vi "NI6071E_HostMain.vi"() -> ()   [LabVIEW 2014, in "NI6071E.lvlib"]
doc: "This VI was developed to test the PH_PPMA_DAQ RT Server Application.\n\nPlease use the PH_PPMA_DAQClient Class within the CS framework."
uses:
  NI6071E.lvlib
  NI6071ECommand.ctl
  NI6071ECommandCluster.ctl
  NI6071EStart.ctl
  NI6071ERead.ctl
  NI6071EConfig.ctl
panel:
  in  "NI6071E DAQ Config RT Client 1":T1={"device (1)"=1, "channels (0)"=["1", "2", "3", "4", "5", "6", "7", "16", "17", "18", "19", "20", "21", "22", "23", "32", "33", "34", "35", "36", "37", "38", "39", "48", "49", "50", "51", "52", "53", "54"], "buffer size (1000 scans)"=1000, "[number of buffers] (1)"=1, "measurement mode structure"={"measurement mode"=0, "reserved"=0}, "input limits (no change)"=[], "coupling & input config (no change:0)"=[{"coupling (no change:0)"=enum."no change", "input config (no change:0)"=1}]} {"measurement mode structure"."measurement mode" items=["no change", "Volts", "Volts RMS", "Ohms", "Diode", "4-wire ohms", "Current", "Current RMS"]; "coupling & input config (no change:0)"."input config (no change:0)" items=["no change", "differential", "ref. single-ended", "non-ref. single-ended", "4-wire"]; "input limits (no change)"."low limit (0.0)" format="%0.2f"; "input limits (no change)"."high limit (0.0)" format="%0.2f"}
  in  "NI6071E DAQ Read":T2={"time limit in sec (-1:auto calculate)"=-1.0, "number of scans to read (-1:all)"=-1} {"time limit in sec (-1:auto calculate)" format="%0.2f"}
  in  "NI6071E DAQ Start":T3={"scan rate (40000 scans/sec)"=1000.0, "trigger type (analog)"=enum."no trigger", "edge or slope \n(rising)"=enum."no change", "number of buffers to acquire (1)"=1, "analog chan (PFI0) & level (2.00)"={"trigger channel (empty)"="", "level (0.0)"=0.0}, "[additional trig params]"={"hysteresis (0.0)"=-1.0, "coupling (no change:0)"=enum."no change", "delay (0 sec)"=0.0, "skip count (0)"=0, "time limit (0 sec)"=0.0}} {"[additional trig params]"."time limit (0 sec)" format="%0.2f"; "[additional trig params]"."delay (0 sec)" format="%0.2f"; "[additional trig params]"."hysteresis (0.0)" format="%0.2f"; "analog chan (PFI0) & level (2.00)"."level (0.0)" format="%0.2f"; "scan rate (40000 scans/sec)" format="%0.2f"}
  out "Measurement":waveform(dbl)[](graph) caption="Measurement data"
  out "RT Error":errorcluster
  in  "NI6071E Command Cluster":T4
  in  "Reset Error":bool
  out "error out":errorcluster
  in  "stop":bool
  out "Response":string
  in  "Connect":bool
  in  "NI6071E DAQ Server":string="apepc01.gsi.de"
  in  "NI6071E Command":T5=enum."CloseConnection"
  in  "Port":u16=6341
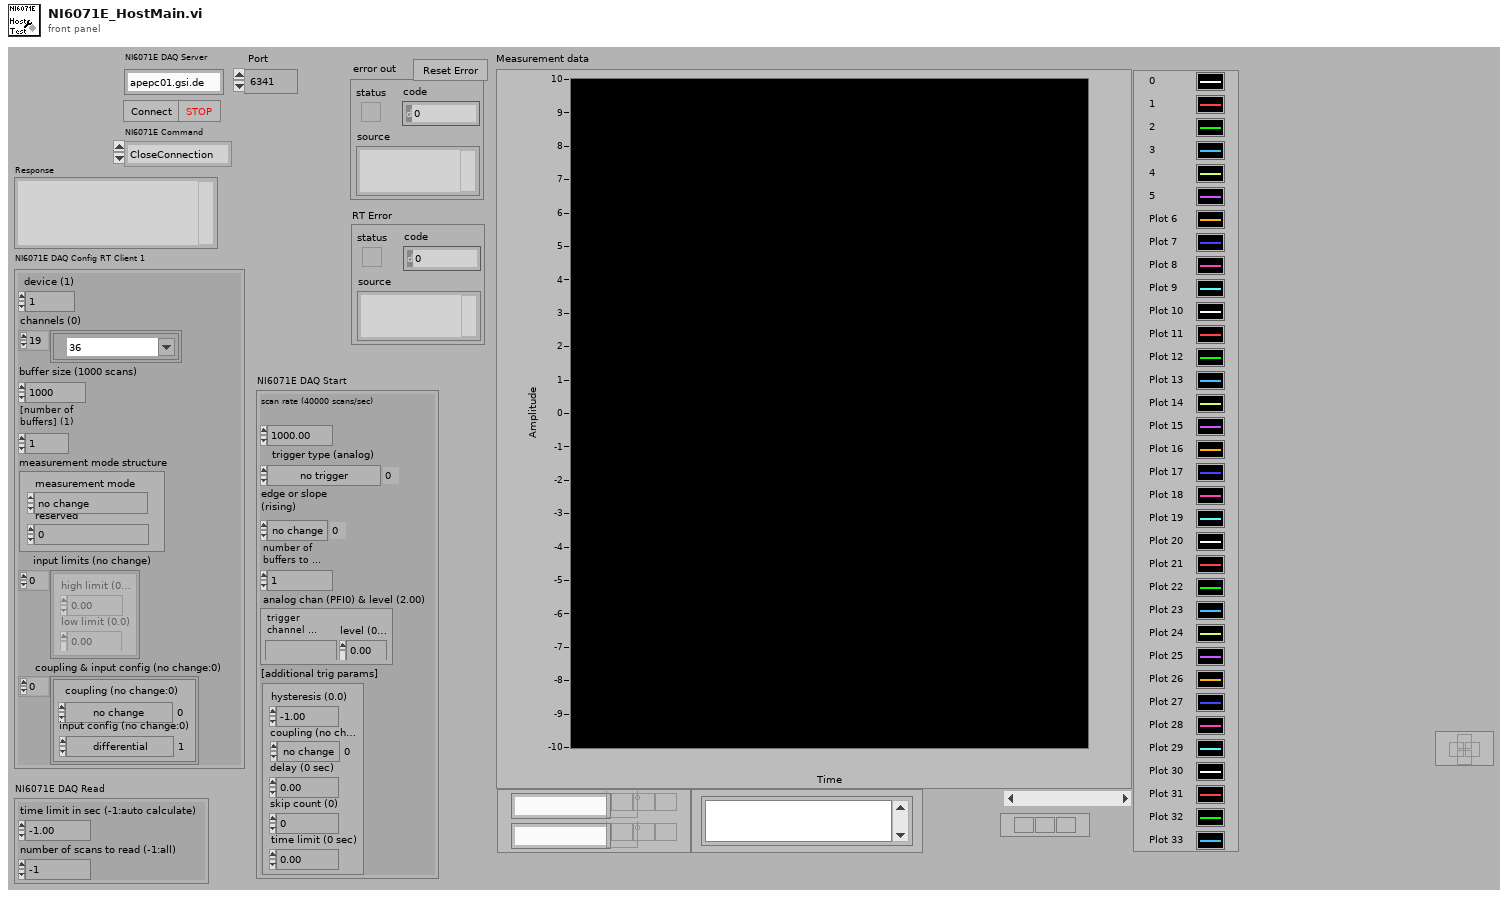
[diagram p1: front panel]
types:
  T1 = typedef "NI6071E.lvlib/NI6071EConfig.ctl" = cluster{"device (1)":i16, "channels (0)":tag[], "buffer size (1000 scans)":i32, "[number of buffers] (1)":i32, "measurement mode structure":cluster{"measurement mode":u16, "reserved":u32}, "input limits (no change)":cluster{"high limit (0.0)":sgl, "low limit (0.0)":sgl}[], "coupling & input config (no change:0)":cluster{"coupling (no change:0)":enum16{"no change", "DC", "AC", "GND", "internal ref."}, "input config (no change:0)":u16}[]}
  T2 = typedef "NI6071E.lvlib/NI6071ERead.ctl" = cluster{"time limit in sec (-1:auto calculate)":sgl, "number of scans to read (-1:all)":i32}
  T3 = typedef "NI6071E.lvlib/NI6071EStart.ctl" = cluster{"scan rate (40000 scans/sec)":sgl, "trigger type (analog)":enum16{"no trigger", "analog", "digital A", "digital A & B", "scan clock gate"}, "edge or slope \n(rising)":enum16{"no change", "rising", "falling"}, "number of buffers to acquire (1)":i32, "analog chan (PFI0) & level (2.00)":cluster{"trigger channel (empty)":string, "level (0.0)":sgl}, "[additional trig params]":cluster{"hysteresis (0.0)":sgl, "coupling (no change:0)":enum16{"no change", "DC", "AC"}, "delay (0 sec)":sgl, "skip count (0)":i32, "time limit (0 sec)":sgl}}
  T4 = typedef "NI6071E.lvlib/NI6071ECommandCluster.ctl" = cluster{"Command":string, "Data":string, "error out":errorcluster}
  T5 = typedef "NI6071E.lvlib/NI6071ECommand.ctl" = enum16{"Ping", "Reset", "ConfigureDAQ", "StartDAQ", "StopDAQ", "GetDAQStatus", "ReadData", "SaveData", "CloseConnection"}
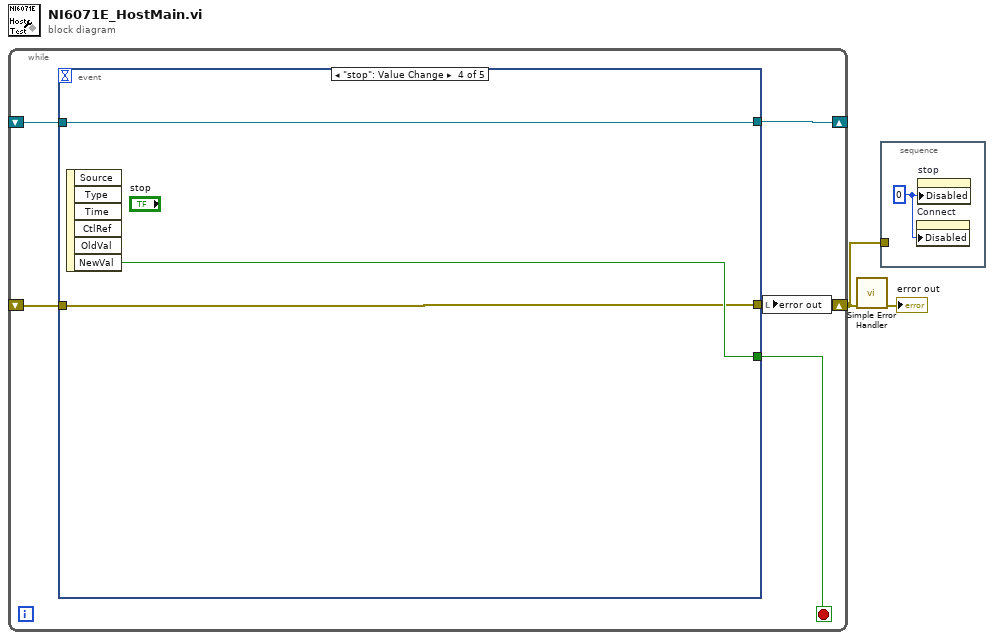
[diagram p0: block diagram]
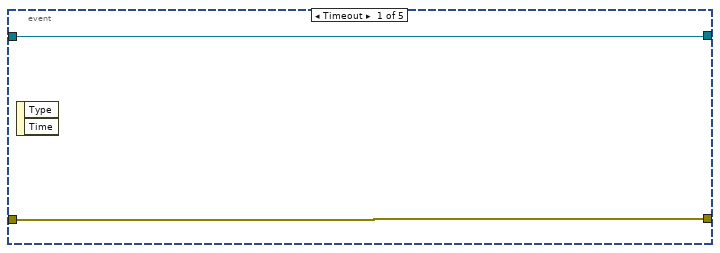
[diagram p2: hidden frame]
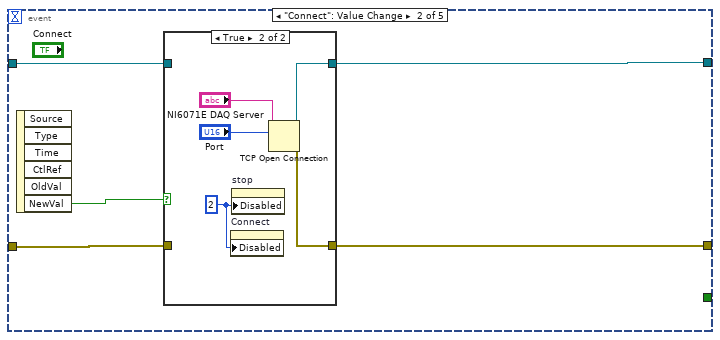
[diagram p3: hidden frame]
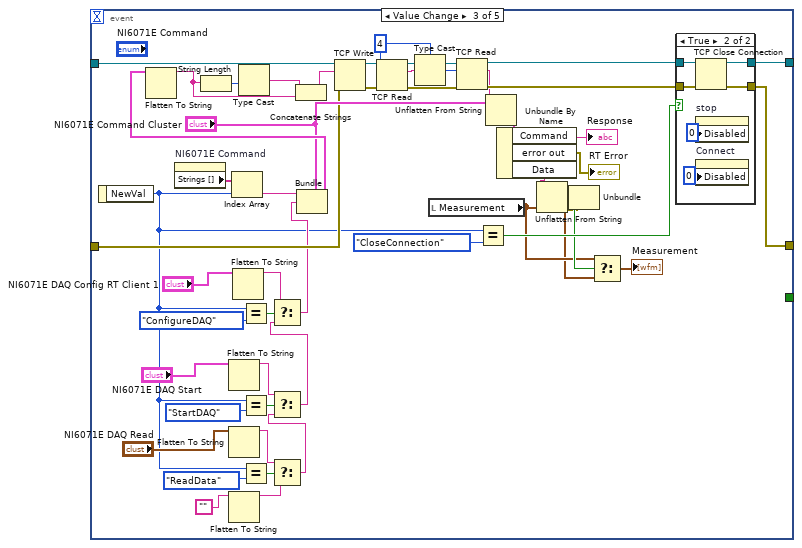
[diagram p5: hidden frame]
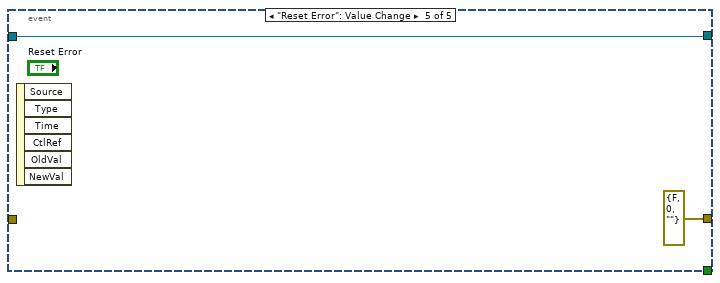
[diagram p7: hidden frame]
diagram:
  n1 = while {
    shift-right: [w6] -> _
    shift-left: _ -> [w7]
    shift-right: [w3] -> w2
    shift-left: _ -> [w5]
    stop <- w4 stop-if-true
    n2 = event shown="[3] \"stop\": Value Change" {
      selector: _ -> [_ _ _ _ _]
      dyn-events: _ -> [_ _ _ _ _]
      timeout: _ -> [_ _ _ _ _]
      tunnel: w7 -> [w8 w13 w72 w81 w85]
      tunnel: [w8 w14 w60 w81 w85] -> w6
      tunnel: [w9 w12 w58 w82 errorcluster {"status"=FALSE, "code"=0, "source"=""} ("error out")] -> w3
      tunnel: w5 -> [w9 w11 w47 w82 _]
      tunnel: [_ _ _ w83 _] -> w4
      event Timeout {
        n3 = event-data() -> ()  [unwired: 1 in, 2 out]
      }
      event "Connect": Value Change {
        n4 = event-data() -> ("NewVal"=w10:bool)  [unwired: 1 in, 5 out]
        n5 = case shown="True" w10 {
          tunnel: [w16 w19] -> w14
          tunnel: w13 -> [w16 _]
          tunnel: [w15 w18] -> w12
          tunnel: w11 -> [w15 _]
          frame False {
          }
          frame True {
            w17 = u8 2 ("Disabled")
            n6 = property on="Connect" class="Bool"("Disabled"=w17) -> ()  [unwired: 2 in, 2 out]
            n7 = property on="stop" class="Bool"("Disabled"=w17) -> ()  [unwired: 2 in, 2 out]
            n8 = TCP Open Connection(address="NI6071E DAQ Server", remote port or service name="Port") -> (connection ID=w19:refnum<k5>, error out=w18:errorcluster)  [unwired: 3 in]
          }
        }
      }
      event Value Change {
        w66 = 4 ("bytes to read")
        n9 = event-data() -> ("NewVal"=w32:T5)  [unwired: 1 in]
        n10 = property on="NI6071E Command" class="Enum (strict)"() -> ("Strings []"=w55:string[])  [unwired: 2 in, 2 out]
        n11 = Flatten To String(anything="NI6071E DAQ Start") -> (data string=w37:string)  [unwired: 3 in, 2 out]
        n12 = Flatten To String(anything="NI6071E DAQ Read") -> (data string=w29:string)  [unwired: 3 in, 2 out]
        n13 = Flatten To String(anything="") -> (data string=w33:string)  [unwired: 3 in, 2 out]
        n14 = Index Array(array=w55, index=w32) -> (element=w53:string)
        n15 = Flatten To String(anything="NI6071E DAQ Config RT Client 1") -> (data string=w41:string)  [unwired: 3 in, 2 out]
        n16 = Equal?(x=w32, y=NI6071ECommand."ConfigureDAQ" ("NewVal")) -> (x = y?=w42:bool)
        n17 = Equal?(x=w32, y=NI6071ECommand."StartDAQ" ("NewVal")) -> (x = y?=w39:bool)
        n18 = Equal?(x=w32, y=NI6071ECommand."ReadData" ("NewVal")) -> (x = y?=w34:bool)
        n19 = Select(t=w29, s=w34, f=w33) -> (s? t:f=w28:string)
        n20 = Select(t=w37, s=w39, f=w28) -> (s? t:f=w36:string)
        n21 = Select(t=w41, s=w42, f=w36) -> (s? t:f=w40:string)
        n22 = Bundle(cluster="NI6071E Command Cluster", "Command"=w53, "Data"=w40) -> (w51:T4)  [unwired: 1 in]
        n23 = Flatten To String(anything=w51) -> (data string=w54:string)  [unwired: 3 in, 2 out]
        n24 = String Length(string=w54) -> (length=w71:i32)
        n25 = Type Cast(x=w71) -> (*(type *) &x=w70:string)  [unwired: 1 in]
        n26 = Concatenate Strings(w70, w54) -> (w69:string)
        n27 = TCP Write(connection ID=w72, data in=w69, error in (no error)=w47) -> (connection ID out=w63:refnum<k5>, error out=w62:errorcluster)  [unwired: 1 in, 1 out]
        n28 = TCP Read(connection ID=w63, bytes to read=w66, error in (no error)=w62) -> (connection ID out=w65:refnum<k5>, data out=w68:string, error out=w64:errorcluster)  [unwired: 2 in]
        n29 = Type Cast(type=w66, x=w68) -> (*(type *) &x=w67:i32)
        n30 = local read "Measurement"() -> (w26:waveform(dbl)[])
        n31 = TCP Read(connection ID=w65, bytes to read=w67, error in (no error)=w64) -> (connection ID out=w61:refnum<k5>, data out=w52:string, error out=w59:errorcluster)  [unwired: 2 in]
        n32 = Equal?(x=w32, y=NI6071ECommand."CloseConnection" ("NewVal")) -> (x = y?=w56:bool)
        n33 = Unflatten From String(type="NI6071E Command Cluster", binary string=w52) -> (value=w49:T4)  [unwired: 3 in, 2 out]
        n34 = Unbundle By Name(w49) -> ("Command"=→"Response":string, "error out"=→"RT Error":errorcluster, "Data"=w45:string)
        n35 = Unflatten From String(type=w26, binary string=w45) -> (value=w24:waveform(dbl)[], error out=w22:errorcluster)  [unwired: 3 in, 1 out]
        n36 = Unbundle(w22) -> ("status"=w27:bool)  [unwired: 2 out]
        n37 = Select(t=w26, s=w27, f=w24) -> (s? t:f=→"Measurement":waveform(dbl)[])
        n38 = case shown="True" w56 {
          tunnel: w61 -> [w74 w80]
          tunnel: [w74 w79] -> w60
          tunnel: w59 -> [w73 w78]
          tunnel: [w73 w77] -> w58
          frame False {
          }
          frame True {
            n39 = TCP Close Connection(connection ID=w80, error in (no error)=w78) -> (connection ID out=w79:refnum<k5>, error out=w77:errorcluster)  [unwired: 1 in]
            n40 = property on="stop" class="Bool"("Disabled"=u8 0) -> ()  [unwired: 2 in, 2 out]
            n41 = property on="Connect" class="Bool"("Disabled"=u8 0) -> ()  [unwired: 2 in, 2 out]
          }
        }
      }
      event "stop": Value Change {
        n42 = event-data() -> ("NewVal"=w83:bool)  [unwired: 1 in, 5 out]
      }
      event "Reset Error": Value Change {
        n43 = event-data() -> ()  [unwired: 1 in, 6 out]
      }
    }
    n44 = local write "error out"(w3) -> ()
  }
  n45 = call <vilib>:"Simple Error Handler.vi"("error in (no error)"=w2) -> ("error out"=→"error out":errorcluster)  [unwired: 4 in, 4 out]
  n46 = stacked-sequence {
    tunnel: w2 -> [_]
    frame #0 {
      w86 = u8 0 ("Disabled")
      n47 = property on="Connect" class="Bool"("Disabled"=w86) -> ()  [unwired: 2 in, 2 out]
      n48 = property on="stop" class="Bool"("Disabled"=w86) -> ()  [unwired: 2 in, 2 out]
    }
  }
